vi "Group Level.vi"(8 "error in (no error)":errorcluster, 11 "Node Ptr":T1 format="%.0x") -> (0 "error out":errorcluster)   [LabVIEW 2024, in "Embedded TDMS Logger System Explorer.lvlib"]
doc: "The Group Page for user definition of the group, allows the user to define the group name and the meta data to be tagged alongside on the group level in the TDMS file.\n\nNote: The Description is not logged in the TDMS file."
uses:
  Embedded TDMS Logger System Explorer.lvlib
  <vilib>/NI VeriStand/Custom Device API/Custom Device Item Ref.ctl
  <vilib>/NI VeriStand/Custom Device API/Set Item Property (Variant).vi
  <vilib>/NI VeriStand/Custom Device API/Get Item Property (Variant).vi
  <vilib>/NI VeriStand/Custom Device API/Custom Device API.lvlib
  Shared/File Classes/Meta Data.ctl
panel:
  in  "Group Level Meta Data":string[][](table)
  in  "Specific Header":cluster{"Section Name":string}={"Section Name"="Specific Page Settings"}
  in  "General Header":cluster{"Section Name":string}={"Section Name"="General Page Settings"}
  in  "Description":string
  in  "Group Name":string
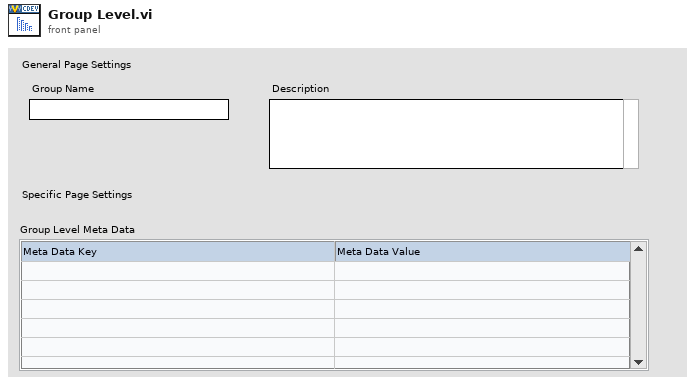
[diagram p1: front panel]
types:
  T1 = typedef "Custom Device API.lvlib/Custom Device Item Ref.ctl" = u64
  T2 = typedef "Meta Data.ctl" = cluster{"Key":string, "Value":string}
  T3 = typedef "Custom Device API.lvlib/Custom Device Item Info.ctl" = cluster{"Name":string, "Is Channel":bool, "GUID":string, "Is Waveform":bool}
  T4 = typedef "Custom Device API.lvlib/Custom Device Commands.ctl" = enum16{"Default", "Item renamed", "Shutdown", "Dynamic button pressed"}
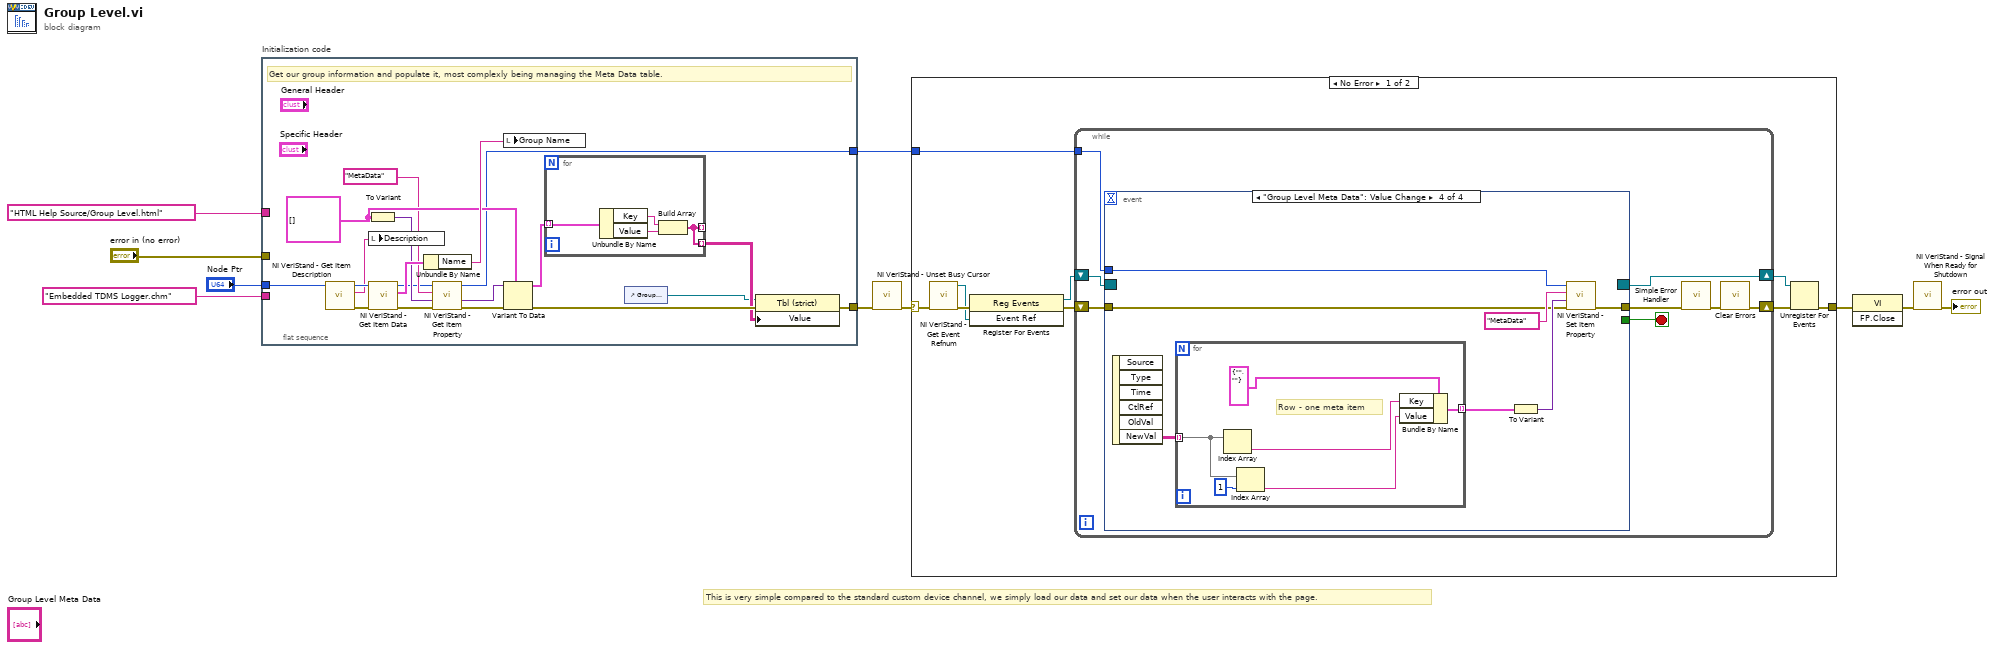
[diagram p0: block diagram]
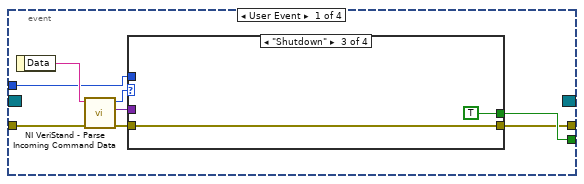
[diagram p2: hidden frame]
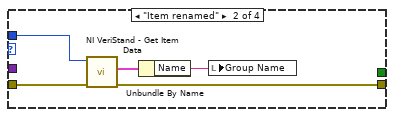
[diagram p4: hidden frame]
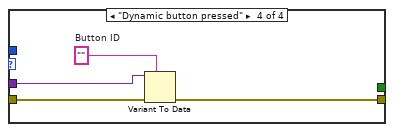
[diagram p5: hidden frame]
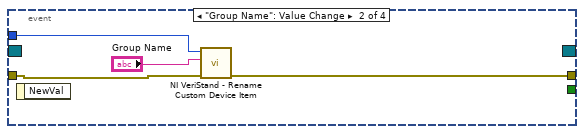
[diagram p6: hidden frame]
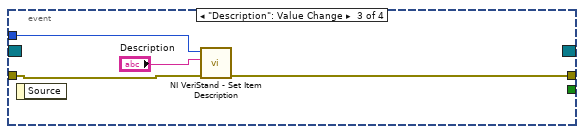
[diagram p7: hidden frame]
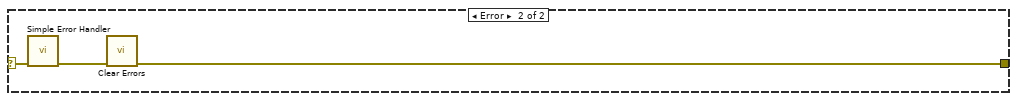
[diagram p8: hidden frame]
diagram:
  # "This is very simple compared to the standard custom device channel, we simply load our data and set our data when the user interacts with the page."
  n1 = flat-sequence "Initialization code" {
    tunnel: "error in (no error)" -> [_]
    tunnel: "Node Ptr" -> [w26]
    tunnel: [w12] -> w6
    tunnel: [w13] -> w3
    tunnel: "HTML Help Source/Group Level.html" ("CD_CHM_Section") -> [_]
    tunnel: "Embedded TDMS Logger.chm" ("CD_CHM_FileName") -> [_]
    frame #0 {
      w17 = T2[] []
      # "Get our group information and populate it, most complexly being managing the Meta Data table."
      n2 = call <vilib>:"NI VeriStand - Get Item Description.vi"("Item Ref in"=w26) -> ("error out"=w28:errorcluster, "Description"=w24:string, "Item Ref out"=w29:T1)  [unwired: 1 in, 7 out]
      n3 = To Variant(anything=w17) -> (Variant=w18:variant)
      n4 = local write "Description"(w24) -> ()
      n5 = call <vilib>:"NI VeriStand - Get Item Data.vi"("error in (no error)"=w28, "Item Ref in"=w29) -> ("error out"=w15:errorcluster, "Item Info"=w27:T3, "Item Ref out"=w14:T1)  [unwired: 7 out]
      n6 = Unbundle By Name(w27) -> ("Name"=w25:string)
      n7 = call-poly <vilib>:"NI VeriStand - Get Item Property.vi"("error in (no error)"=w15, "Default Value"=w18, "Property Name"="MetaData", "Item Ref in"=w14) -> ("error out"=w19:errorcluster, "Value"=w20:variant, "Item Ref out"=w13:T1)  [unwired: 4 in, 1 out]
      n8 = local write "Group Name"(w25) -> ()
      n9 = Variant To Data(error in=w19, type=w17, Variant=w20) -> (data=w21:T2[], error out=w23:errorcluster)
      n10 = for {
        tunnel: w21 -> [w33] mode=indexing
        tunnel: [w30] -> _ mode=indexing
        tunnel: [w30] -> w22 mode=indexing
        n11 = Unbundle By Name(w33) -> ("Key"=w32:string, "Value"=w31:string)
        n12 = Build Array(w32, w31) -> (w30:string[])
      }
      n13 = control-ref of="Group Level Meta Data"() -> (w11:refnum<vi>)
      n14 = property class="Tbl (strict)"(reference=w11, error in=w23, "Value"=w22) -> (error out=w12:errorcluster)  [unwired: 1 out]
    }
  }
  n15 = call <vilib>:"NI VeriStand - Unset Busy Cursor.vi"("error in (no error)"=w6) -> ("error out"=w5:errorcluster)  [unwired: 10 out]
  n16 = case shown="No Error" w5 {
    selector: w5 -> [w34 w94]
    tunnel: [w39 w92] -> w10
    tunnel: w3 -> [w35 _]
    frame No Error {
      n17 = call <vilib>:"NI VeriStand - Get Event Refnum.vi"("error in (no error)"=w34) -> ("error out"=w42:errorcluster, "Event Ref"=w38:refnum<user-event>)  [unwired: 9 out]
      n18 = register-events(error in=w42, w38) -> (reference out=w36:refnum<event-registration>, error out=w37:errorcluster)  [unwired: 1 in]
      n19 = while {
        tunnel: w35 -> [w46]
        shift-right: [w43] -> w40
        shift-left: w37 -> [w49]
        shift-right: [w50] -> w41
        shift-left: w36 -> [w48]
        stop <- w47 stop-if-true
        n20 = event shown="[3] \"Group Level Meta Data\": Value Change" {
          selector: w48 -> [_ _ _ _]
          dyn-events: [_ _ _ _] -> w50
          timeout: _ -> [_ _ _ _]
          tunnel: w49 -> [w58 w74 w77 w80]
          tunnel: [w54 _ _ _] -> w47
          tunnel: [w53 w73 w76 w79] -> w45
          tunnel: w46 -> [w52 w72 w78 w81]
          event User Event {
            n21 = event-data() -> ("Data"=w57:string)  [unwired: 1 out]
            n22 = call <vilib>:"NI VeriStand - Parse Incoming Command Data.vi"("error in (no error)"=w58, "Incoming data"=w57) -> ("error out"=w56:errorcluster, "Outgoing data"=w51:variant, "Action"=w55:T4)  [unwired: 7 out]
            n23 = case shown="\"Shutdown\"" w55 {
              tunnel: w56 -> [w59 w64 w65 w70]
              tunnel: [_ _ TRUE _] -> w54
              tunnel: [w59 w61 w65 w67] -> w53
              tunnel: w52 -> [_ w63 _ _]
              tunnel: w51 -> [_ _ _ w69]
              frame "Default", Default {
              }
              frame "Item renamed" {
                n24 = call <vilib>:"NI VeriStand - Get Item Data.vi"("error in (no error)"=w64, "Item Ref in"=w63) -> ("error out"=w61:errorcluster, "Item Info"=w62:T3)  [unwired: 8 out]
                n25 = Unbundle By Name(w62) -> ("Name"=w60:string)
                n26 = local write "Group Name"(w60) -> ()
              }
              frame "Shutdown" {
              }
              frame "Dynamic button pressed" {
                w68 = ""  # Button ID
                n27 = Variant To Data(error in=w70, type=w68, Variant=w69) -> (error out=w67:errorcluster)  [unwired: 1 out]
              }
            }
          }
          event "Group Name": Value Change {
            n28 = event-data() -> ()  [unwired: 2 out]
            n29 = call <vilib>:"NI VeriStand - Rename Custom Device Item.vi"("error in (no error)"=w74, "New Name"="Group Name", "Item Ref in"=w72) -> ("error out"=w73:errorcluster)  [unwired: 1 in, 7 out]
          }
          event "Description": Value Change {
            n30 = event-data() -> ()  [unwired: 2 out]
            n31 = call <vilib>:"NI VeriStand - Set Item Description.vi"("error in (no error)"=w77, "Description"="Description", "Item Ref in"=w78) -> ("error out"=w76:errorcluster)  [unwired: 8 out]
          }
          event "Group Level Meta Data": Value Change {
            n32 = event-data() -> ("NewVal"=w85:string[][])  [unwired: 6 out]
            n33 = for {
              tunnel: w85 -> [w90] mode=indexing
              tunnel: [w87] -> w84 mode=indexing
              # "Row - one meta item"
              n34 = Index Array(array=w90) -> (element=w88:string)  [unwired: 1 in]
              n35 = Index Array(array=w90, index=1) -> (element=w89:string)
              n36 = Bundle By Name(cluster=T2 {"Key"="", "Value"=""} ("Meta Data"), "Key"=w88, "Value"=w89) -> (w87:T2)
            }
            n37 = To Variant(anything=w84) -> (Variant=w83:variant)
            n38 = call-poly <vilib>:"NI VeriStand - Set Item Property.vi"("error in (no error)"=w80, "Value"=w83, "Property Name"="MetaData", "Item Ref in"=w81) -> ("error out"=w79:errorcluster)  [unwired: 5 in, 2 out]
          }
        }
        n39 = call <vilib>:"Simple Error Handler.vi"("error in (no error)"=w45) -> ("error out"=w44:errorcluster)  [unwired: 1 in, 7 out]
        n40 = call <vilib>:"Clear Errors.vi"("error in (no error)"=w44) -> ("error out"=w43:errorcluster)  [unwired: 1 in, 5 out]
      }
      n41 = Unregister For Events(event registration refnum=w41, error in=w40) -> (error out=w39:errorcluster)
    }
    frame Error {
      n42 = call <vilib>:"Simple Error Handler.vi"("error in (no error)"=w94) -> ("error out"=w93:errorcluster)  [unwired: 1 in, 7 out]
      n43 = call <vilib>:"Clear Errors.vi"("error in (no error)"=w93) -> ("error out"=w92:errorcluster)  [unwired: 1 in, 5 out]
    }
  }
  n44 = invoke class="VI" method="FP.Close"(error in=w10) -> (error out=w9:errorcluster)  [unwired: 2 in, 2 out]
  n45 = call <vilib>:"NI VeriStand - Signal When Ready for Shutdown.vi"("error in (no error)"=w9) -> ("error out"=→"error out":errorcluster)  [unwired: 10 out]
